vi "GT Get Di Raw.vi"(8 "error in (no error)":errorcluster caption="错误输入（无错误）", 9 "pValue":i32, 10 "diType":i16, 11 "cardNum":i16) -> (0 "error out":errorcluster caption="错误输出", 1 "pValue out":i32, 3 "function return":i16)   [LabVIEW 2020, in "gts.lvlib"]
doc: "GT_API GT_GetDiRaw(short cardNum,short diType,long *pValue);"
uses:
  gts.lvlib
  dll/32bit/multi_card/gts.dll
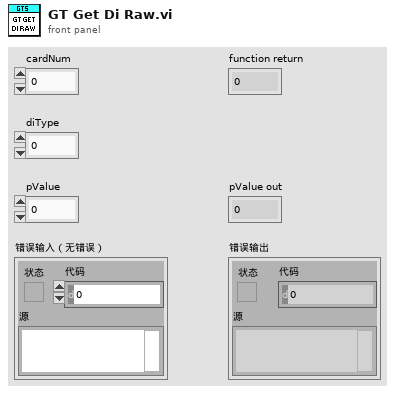
[diagram p1: front panel]
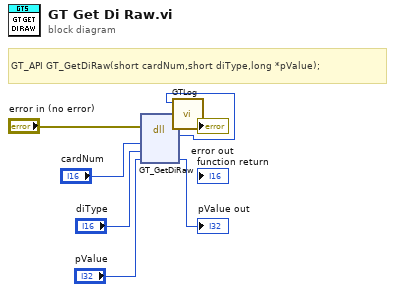
[diagram p0: block diagram]
diagram:
  # "GT_API GT_GetDiRaw(short cardNum,short diType,long *pValue);"
  n1 = dll-call lib="C:/1228/dll/32bit/multi_card/gts.dll" fn="GT_GetDiRaw"(error in="error in (no error)", "cardNum"="cardNum", "diType"="diType", "pValue"="pValue") -> (error out=w3:errorcluster, w1:i16, "pValue"=→"pValue out":i32)  [unwired: 4 in, 1 out]
  n2 = call "GTLog.vi"("error in (no error)"=w3, "Numeric"=w1) -> ("error out"=→"error out":errorcluster)  [unwired: 9 in]
